vi "Write outgoing label data.vi"(4 "ScheduledSDI":bool, 6 "Iteration":i32, 8 "error in (no error)":errorcluster, 9 "Last iteration values":dbl[](array[numeric]), 10 "This iteration values":dbl[](array[numeric]), 11 "Label Settings":T1 {"Words"."Param Setting"."Num Bits" min=1 max=32; "Words"."Param Setting"."Start Bit" min=8 max=31; "Words"."Block Data Refs"."Data Reference" format="%.0x"; "Label" format="%.0o"}) -> (0 "error out":errorcluster, 1 "Last iteration values Out":dbl[](array[numeric]), 3 "Label Settings":T1 {"Words"."Param Setting"."Num Bits" min=1 max=32; "Words"."Param Setting"."Start Bit" min=8 max=31; "Words"."Block Data Refs"."Data Reference" format="%.0x"; "Label" format="%.0o"})   [LabVIEW 2012, in "AIT 429 Engine.lvlib"]
uses:
  AIT 429 Engine.lvlib
  RT Controls/RT Label Settings.ctl
  Shared/Controls and Global/Label.ctl
  Shared/Controls and Global/transferPeriod.ctl
  RT Controls/Driver Data.ctl
  RT Controls/RT Word Settings.ctl
  <vilib>/NI Veristand/Custom Device API/Block Data Reference.ctl
  <vilib>/NI Veristand/Custom Device API/Data Reference.ctl
  RT Controls/RT Param Setting.ctl
  Shared/Controls and Global/Start Bit.ctl
  Shared/Controls and Global/Number of Bits.ctl
  Shared/Controls and Global/TransferType.ctl
  <instrlib>/AIT 429/AIT 429.lvlib
  ARINC 429 Shared.lvlib
  <vilib>/NI Veristand/Custom Device API/Custom Device API.lvlib
panel:
  in  "Array length":i32
  in  "Array index":i32
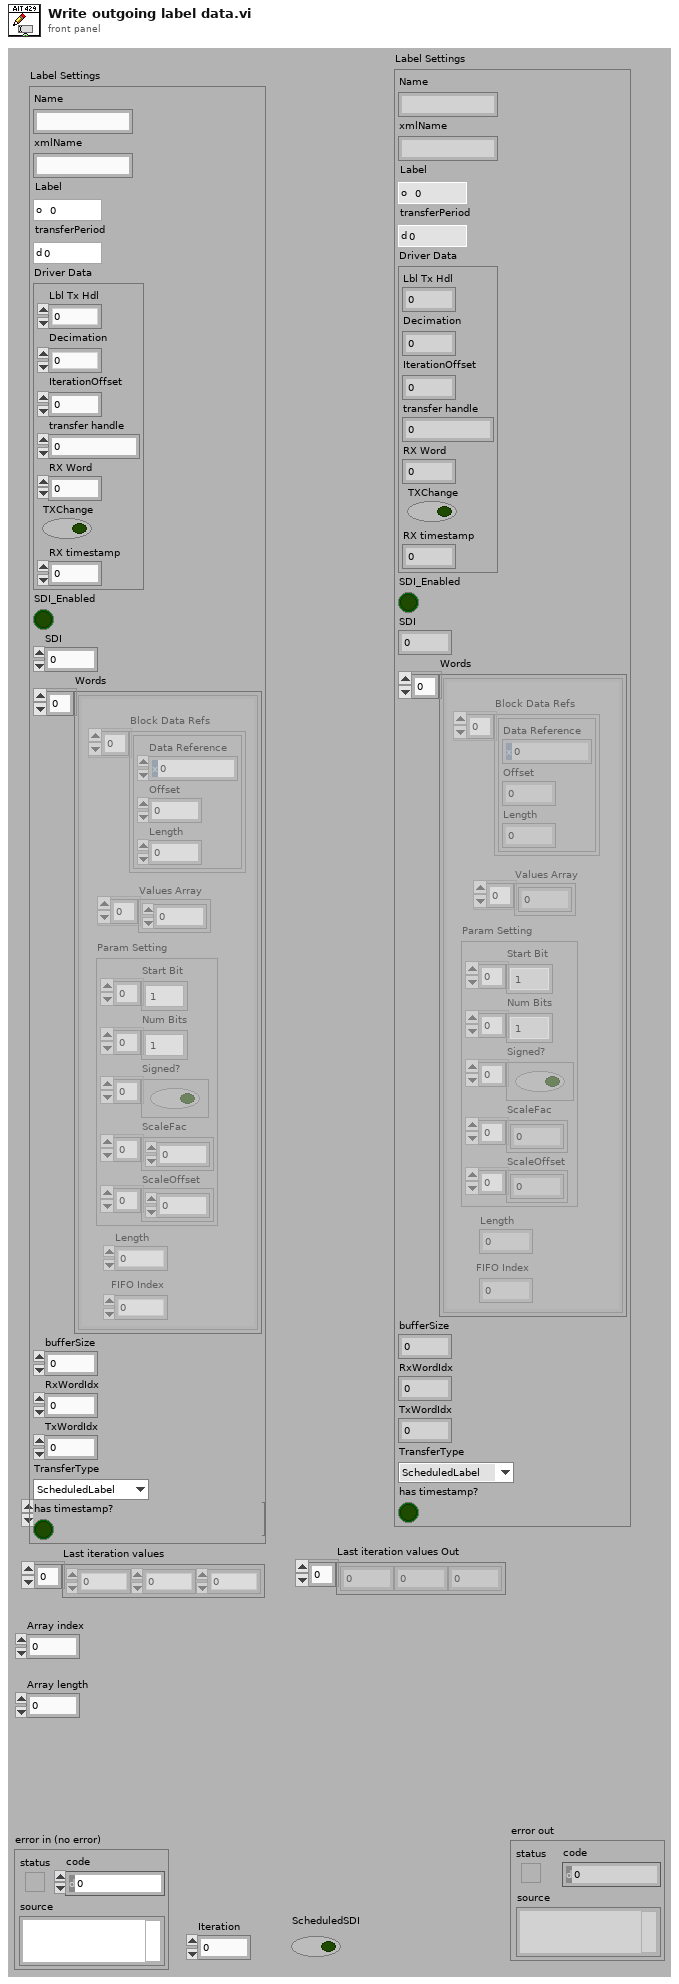
[diagram p1: front panel]
types:
  T1 = typedef "AIT 429 Engine.lvlib/RT Label Settings.ctl" = cluster{"Name":string, "xmlName":string, "Label":T2, "transferPeriod":T3, "Driver Data":T4, "SDI_Enabled":bool, "SDI":u8, "Words":T5[], "bufferSize":u32, "RxWordIdx":i32, "TxWordIdx":i32, "TransferType":T11, "has timestamp?":bool}
  T2 = typedef "ARINC 429 Shared.lvlib/Label.ctl" = u8
  T3 = typedef "ARINC 429 Shared.lvlib/transferPeriod.ctl" = u32
  T4 = typedef "AIT 429 Engine.lvlib/Driver Data.ctl" = cluster{"Lbl Tx Hdl":u32, "Decimation":i32, "IterationOffset":i32, "transfer handle":u32, "RX Word":u32, "TXChange":bool, "RX timestamp":dbl}
  T5 = typedef "AIT 429 Engine.lvlib/RT Word Settings.ctl" = cluster{"Block Data Refs":T6[], "Values Array":dbl[], "Length":i32, "FIFO Index":i32, "Param Setting":T8}
  T6 = typedef "Custom Device API.lvlib/Block Data Reference.ctl" = cluster{"Data Reference":T7, "Offset":i32, "Length":i32}
  T7 = typedef "Custom Device API.lvlib/Data Reference.ctl" = i32
  T8 = typedef "AIT 429 Engine.lvlib/RT Param Setting.ctl" = cluster{"Start Bit":T9[], "Num Bits":T10[], "Signed?":bool[], "ScaleFac":dbl[], "ScaleOffset":dbl[]}
  T9 = typedef "ARINC 429 Shared.lvlib/Start Bit.ctl" = i32
  T10 = typedef "ARINC 429 Shared.lvlib/Number of Bits.ctl" = i32
  T11 = typedef "ARINC 429 Shared.lvlib/TransferType.ctl" = enum16{"ScheduledLabel", "Acyclic", "Block", "Strobe"}
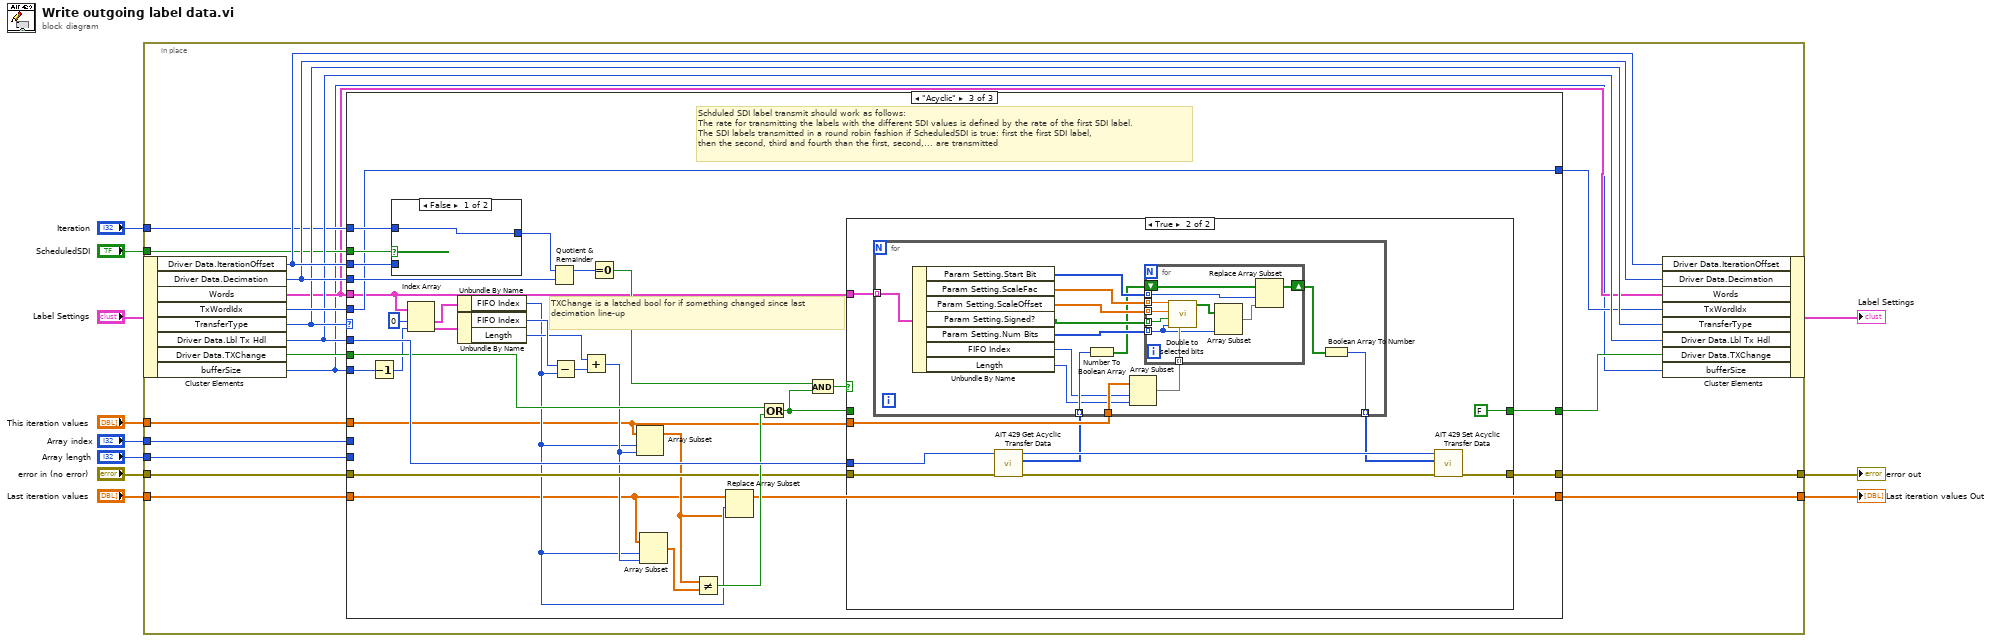
[diagram p0: block diagram]
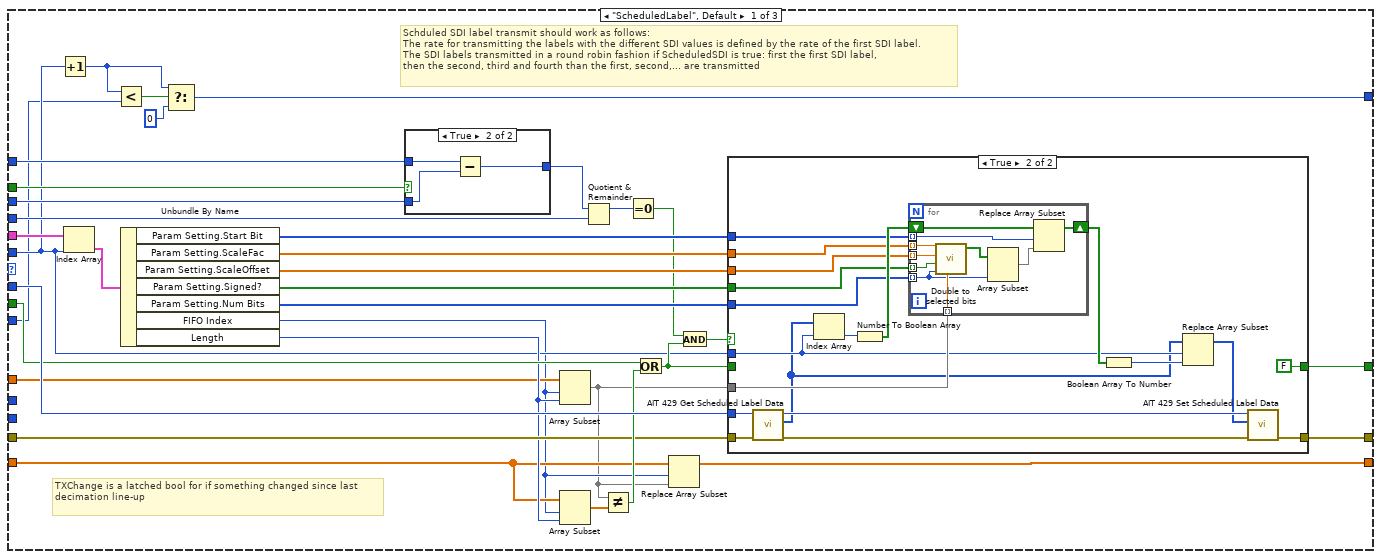
[diagram p2: hidden frame]
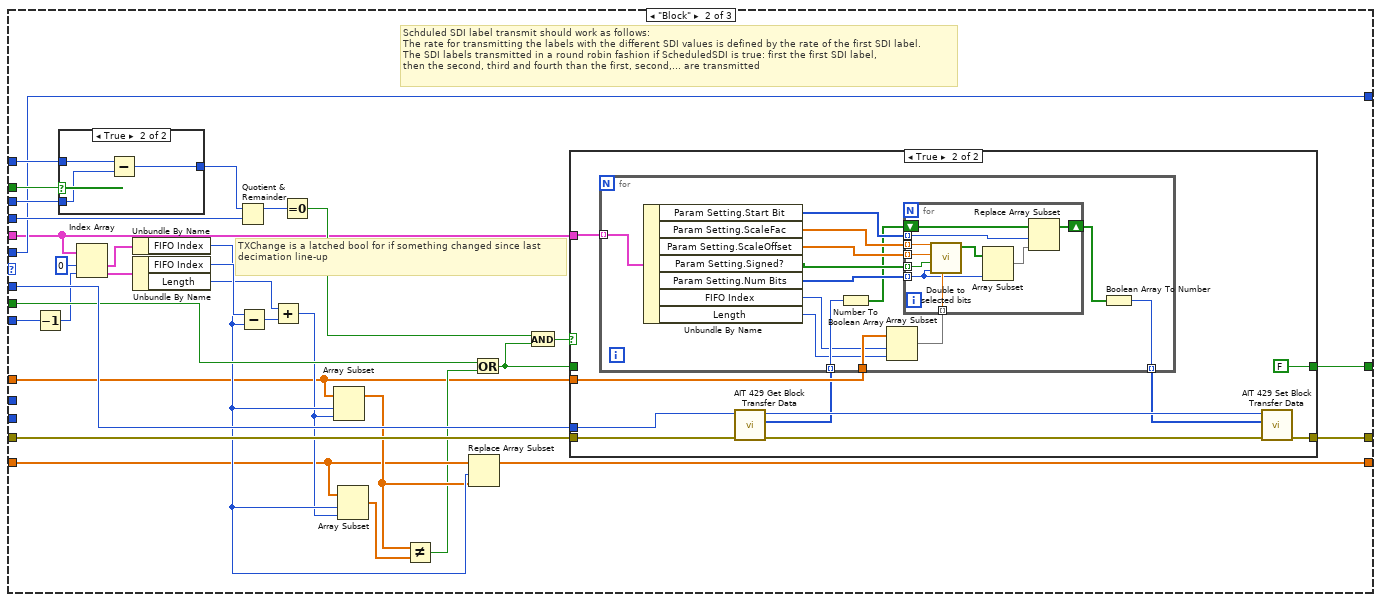
[diagram p5: hidden frame]
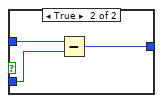
[diagram p9: hidden frame]
diagram:
  n1 = in-place {
    in-place-border: "This iteration values" -> [w27]
    in-place-border: "Array index" -> [w26]
    in-place-border: "Array length" -> [w25]
    in-place-border: "error in (no error)" -> [w24]
    in-place-border: "Last iteration values" -> [w23]
    in-place-border: [w22] -> w5
    in-place-border: "Iteration" -> [w17]
    in-place-border: "ScheduledSDI" -> [w16]
    in-place-border: [w13] -> w1
    n2 = in-place-cluster #1("Label Settings") -> ("Driver Data.IterationOffset"=w21:i32, "Driver Data.Decimation"=w20:i32, "Words"=w14:T5[], "TxWordIdx"=w30:i32, "TransferType"=w19:T11, "Driver Data.Lbl Tx Hdl"=w18:u32, "Driver Data.TXChange"=w29:bool, "bufferSize"=w12:u32)
    n3 = case shown="\"Acyclic\"" w19 {
      tunnel: w30 -> [w36 w118 w189]
      tunnel: w14 -> [w65 w117 w188]
      tunnel: w21 -> [w64 w132 w204]
      tunnel: w20 -> [w63 w131 w203]
      tunnel: w18 -> [w62 w130 w202]
      tunnel: w29 -> [w61 w129 w201]
      tunnel: [w60 w128 w200] -> w28
      tunnel: w27 -> [w38 w101 w173]
      tunnel: w26 -> [_ _ _]
      tunnel: w25 -> [_ _ _]
      tunnel: w24 -> [w47 w122 w193]
      tunnel: w23 -> [w34 w104 w174]
      tunnel: [w46 w121 w192] -> w22
      tunnel: w17 -> [w45 w120 w191]
      tunnel: w16 -> [w44 w119 w190]
      tunnel: [w41 w118 w189] -> w15
      tunnel: [w35 w108 w178] -> w13
      tunnel: w12 -> [w31 w115 w186]
      frame "ScheduledLabel", Default {
        # "TXChange is a latched bool for if something changed since last decimation line-up"
        # "Schduled SDI label transmit should work as follows:\nThe rate for transmitting the labels with the different SDI values is defined by the rate of the first SDI label.\nThe SDI labels transmitted in a round robin fashion if ScheduledSDI is true: first the first SDI label, \nthen the second, third and fourth than the first, second,... are transmitted"
        n4 = Increment(x=w36) -> (x+1=w39:i32)
        n5 = Index Array(array=w65, index=w36) -> (element=w59:T5)
        n6 = Less?(x=w39, y=w31) -> (x < y?=w43:bool)
        n7 = Unbundle By Name(w59) -> ("Param Setting.Start Bit"=w58:T9[], "Param Setting.ScaleFac"=w57:dbl[], "Param Setting.ScaleOffset"=w56:dbl[], "Param Setting.Signed?"=w55:bool[], "Param Setting.Num Bits"=w54:T10[], "FIFO Index"=w33:i32, "Length"=w40:i32)
        n8 = Select(t=w39, s=w43, f=0 ("TxWordIdx")) -> (s? t:f=w41:i32)
        n9 = case shown="True" w44 {
          tunnel: w45 -> [w97 w98]
          tunnel: [w97 w100] -> w52
          tunnel: w64 -> [_ w99]
          frame False {
          }
          frame True {
            n10 = Subtract(x=w98, y=w99) -> (x-y=w100:i32)
          }
        }
        n11 = Array Subset(array=w38, index=w33, length=w40) -> (w32:dbl[])
        n12 = Array Subset(array=w34, index=w33, length=w40) -> (w37:dbl[])
        n13 = Quotient & Remainder(x=w52, y=w63) -> (x-y*floor(x/y)=w53:i32)  [unwired: 1 out]
        n14 = Not Equal?(x=w32, y=w37) -> (x != y?=w51:bool)
        n15 = Equal To 0?(x=w53) -> (x = 0?=w50:bool)
        n16 = Or(x=w61, y=w51) -> (x .or. y?=w48:bool)
        n17 = Replace Array Subset(array=w34, new element=w32, index=w33) -> (w35:dbl[])
        n18 = And(x=w50, y=w48) -> (x .and. y?=w49:bool)
        n19 = case shown="True" w49 {
          tunnel: w58 -> [_ w83]
          tunnel: w54 -> [_ w84]
          tunnel: [w67 w74] -> w46
          tunnel: w47 -> [w67 w78]
          tunnel: w62 -> [_ w77]
          tunnel: w57 -> [_ w82]
          tunnel: w56 -> [_ w81]
          tunnel: w55 -> [_ w80]
          tunnel: w32 -> [_ w79]
          tunnel: w48 -> [w66 _]
          tunnel: [w66 FALSE] -> w60
          tunnel: w36 -> [_ w71]
          frame False {
          }
          frame True {
            (unwired) FALSE
            n20 = call <instrlib>:"AIT 429 Get Scheduled Label Data.vi"("error in (no error)"=w78, "scheduled label handle"=w77) -> ("error out"=w75:errorcluster, "word array"=w70:u32[], "scheduled label handle"=w73:u32)  [unwired: 7 in]
            n21 = Index Array(array=w70, index=w71) -> (element=w76:u32)
            n22 = Number To Boolean Array(number=w76) -> (Boolean array=w86:bool[])
            n23 = for {
              tunnel: w83 -> [w95] mode=indexing
              tunnel: w84 -> [w90] mode=indexing
              tunnel: w79 -> [w91] mode=indexing
              shift-right: [w93] -> w85
              shift-left: w86 -> [w96]
              tunnel: w82 -> [w89] mode=indexing
              tunnel: w81 -> [w88] mode=indexing
              tunnel: w80 -> [w87] mode=indexing
              n24 = call "Double to selected bits.vi"("Double"=w91, "Number of Bits"=w90, "Signed?"=w87, "ScaleOffset"=w88, "ScaleFac"=w89) -> ("Bits"=w92:bool[])  [unwired: 6 in]
              n25 = Array Subset(array=w92, length=w90) -> (w94:bool[])  [unwired: 1 in]
              n26 = Replace Array Subset(array=w96, new element=w94, index=w95) -> (w93:bool[])
            }
            n27 = Boolean Array To Number(Boolean array=w85) -> (number=w72:u32)
            n28 = Replace Array Subset(array=w70, new element=w72, index=w71) -> (w69:u32[])
            n29 = call <instrlib>:"AIT 429 Set Scheduled Label Data.vi"("error in (no error)"=w75, "word array"=w69, "scheduled label handle"=w73) -> ("error out"=w74:errorcluster)  [unwired: 6 in, 2 out]
          }
        }
      }
      frame "Block" {
        # "TXChange is a latched bool for if something changed since last decimation line-up"
        # "Schduled SDI label transmit should work as follows:\nThe rate for transmitting the labels with the different SDI values is defined by the rate of the first SDI label.\nThe SDI labels transmitted in a round robin fashion if ScheduledSDI is true: first the first SDI label, \nthen the second, third and fourth than the first, second,... are transmitted"
        n30 = Decrement(x=w115) -> (x-1=w114:u32)
        n31 = case shown="True" w119 {
          tunnel: w120 -> [w169 w170]
          tunnel: [w169 w172] -> w126
          tunnel: w132 -> [_ w171]
          frame False {
          }
          frame True {
            n32 = Subtract(x=w170, y=w171) -> (x-y=w172:i32)
          }
        }
        n33 = Index Array(array=w117, index #1=0 ("index"), index #2=w114) -> (element #1=w113:T5, element #2=w112:T5)
        n34 = Unbundle By Name(w113) -> ("FIFO Index"=w107:i32)
        n35 = Unbundle By Name(w112) -> ("FIFO Index"=w111:i32, "Length"=w109:i32)
        n36 = Quotient & Remainder(x=w126, y=w131) -> (x-y*floor(x/y)=w127:i32)  [unwired: 1 out]
        n37 = Subtract(x=w111, y=w107) -> (x-y=w110:i32)
        n38 = Add(x=w109, y=w110) -> (x+y=w106:i32)
        n39 = Equal To 0?(x=w127) -> (x = 0?=w125:bool)
        n40 = Array Subset(array=w101, index=w107, length=w106) -> (w105:dbl[])
        n41 = Array Subset(array=w104, index=w107, length=w106) -> (w103:dbl[])
        n42 = Not Equal?(x=w105, y=w103) -> (x != y?=w102:bool)
        n43 = Replace Array Subset(array=w104, new element=w105, index=w107) -> (w108:dbl[])
        n44 = Or(x=w129, y=w102) -> (x .or. y?=w123:bool)
        n45 = And(x=w125, y=w123) -> (x .and. y?=w124:bool)
        n46 = case shown="True" w124 {
          tunnel: [w134 w139] -> w121
          tunnel: w122 -> [w134 w141]
          tunnel: w130 -> [_ w138]
          tunnel: w101 -> [_ w142]
          tunnel: w123 -> [w133 _]
          tunnel: [w133 FALSE] -> w128
          tunnel: w117 -> [_ w143]
          frame False {
          }
          frame True {
            n47 = call <instrlib>:"AIT 429 Get Block Transfer Data.vi"("error in"=w141, "block transfer handle in"=w138) -> ("error out"=w140:errorcluster, "word array out"=w136:u32[], "block transfer handle out"=w137:u32)  [unwired: 7 in]
            n48 = for {
              tunnel: w142 -> [w148]
              tunnel: [w157] -> w135 mode=indexing
              tunnel: w143 -> [w151] mode=indexing
              tunnel: w136 -> [w149] mode=indexing
              n49 = Unbundle By Name(w151) -> ("Param Setting.Start Bit"=w156:T9[], "Param Setting.ScaleFac"=w155:dbl[], "Param Setting.ScaleOffset"=w154:dbl[], "Param Setting.Signed?"=w153:bool[], "Param Setting.Num Bits"=w152:T10[], "FIFO Index"=w147:i32, "Length"=w146:i32)
              n50 = Number To Boolean Array(number=w149) -> (Boolean array=w150:bool[])
              n51 = Array Subset(array=w148, index=w147, length=w146) -> (w145:dbl[])
              n52 = for {
                tunnel: w156 -> [w167] mode=indexing
                tunnel: w152 -> [w162] mode=indexing
                tunnel: w145 -> [w163] mode=indexing
                shift-right: [w165] -> w158
                shift-left: w150 -> [w168]
                tunnel: w155 -> [w161] mode=indexing
                tunnel: w154 -> [w160] mode=indexing
                tunnel: w153 -> [w159] mode=indexing
                n53 = call "Double to selected bits.vi"("Double"=w163, "Number of Bits"=w162, "Signed?"=w159, "ScaleOffset"=w160, "ScaleFac"=w161) -> ("Bits"=w164:bool[])  [unwired: 6 in]
                n54 = Array Subset(array=w164, length=w162) -> (w166:bool[])  [unwired: 1 in]
                n55 = Replace Array Subset(array=w168, new element=w166, index=w167) -> (w165:bool[])
              }
              n56 = Boolean Array To Number(Boolean array=w158) -> (number=w157:u32)
            }
            n57 = call <instrlib>:"AIT 429 Set Block Transfer Data.vi"("error in (no error)"=w140, "word array"=w135, "block transfer handle in"=w137) -> ("error out"=w139:errorcluster)  [unwired: 6 in, 2 out]
          }
        }
      }
      frame "Acyclic" {
        # "TXChange is a latched bool for if something changed since last decimation line-up"
        # "Schduled SDI label transmit should work as follows:\nThe rate for transmitting the labels with the different SDI values is defined by the rate of the first SDI label.\nThe SDI labels transmitted in a round robin fashion if ScheduledSDI is true: first the first SDI label, \nthen the second, third and fourth than the first, second,... are transmitted"
        n58 = Decrement(x=w186) -> (x-1=w185:u32)
        n59 = case shown="False" w190 {
          tunnel: w191 -> [w241 w242]
          tunnel: [w241 w244] -> w198
          tunnel: w204 -> [_ w243]
          frame False {
          }
          frame True {
            n60 = Subtract(x=w242, y=w243) -> (x-y=w244:i32)
          }
        }
        n61 = Index Array(array=w188, index #1=0 ("index"), index #2=w185) -> (element #1=w184:T5, element #2=w183:T5)
        n62 = Unbundle By Name(w184) -> ("FIFO Index"=w177:i32)
        n63 = Unbundle By Name(w183) -> ("FIFO Index"=w182:i32, "Length"=w180:i32)
        n64 = Quotient & Remainder(x=w198, y=w203) -> (x-y*floor(x/y)=w199:i32)  [unwired: 1 out]
        n65 = Subtract(x=w182, y=w177) -> (x-y=w181:i32)
        n66 = Add(x=w180, y=w181) -> (x+y=w179:i32)
        n67 = Equal To 0?(x=w199) -> (x = 0?=w196:bool)
        n68 = Array Subset(array=w173, index=w177, length=w179) -> (w176:dbl[])
        n69 = Array Subset(array=w174, index=w177, length=w179) -> (w175:dbl[])
        n70 = Not Equal?(x=w176, y=w175) -> (x != y?=w197:bool)
        n71 = Replace Array Subset(array=w174, new element=w176, index=w177) -> (w178:dbl[])
        n72 = Or(x=w201, y=w197) -> (x .or. y?=w194:bool)
        n73 = And(x=w196, y=w194) -> (x .and. y?=w195:bool)
        n74 = case shown="True" w195 {
          tunnel: [w206 w208] -> w192
          tunnel: w193 -> [w206 w210]
          tunnel: w202 -> [_ w213]
          tunnel: w173 -> [_ w214]
          tunnel: w194 -> [w205 _]
          tunnel: [w205 FALSE] -> w200
          tunnel: w188 -> [_ w215]
          frame False {
          }
          frame True {
            n75 = call <instrlib>:"AIT 429 Get Acyclic Transfer Data.vi"("error in (no error)"=w210, "transfer handle"=w213) -> ("error out"=w209:errorcluster, "word array"=w211:u32[], "transfer handle"=w212:u32)  [unwired: 7 in]
            n76 = for {
              tunnel: w214 -> [w220]
              tunnel: [w229] -> w207 mode=indexing
              tunnel: w215 -> [w223] mode=indexing
              tunnel: w211 -> [w221] mode=indexing
              n77 = Unbundle By Name(w223) -> ("Param Setting.Start Bit"=w228:T9[], "Param Setting.ScaleFac"=w227:dbl[], "Param Setting.ScaleOffset"=w226:dbl[], "Param Setting.Signed?"=w225:bool[], "Param Setting.Num Bits"=w224:T10[], "FIFO Index"=w219:i32, "Length"=w218:i32)
              n78 = Number To Boolean Array(number=w221) -> (Boolean array=w222:bool[])
              n79 = Array Subset(array=w220, index=w219, length=w218) -> (w217:dbl[])
              n80 = for {
                tunnel: w228 -> [w239] mode=indexing
                tunnel: w224 -> [w234] mode=indexing
                tunnel: w217 -> [w235] mode=indexing
                shift-right: [w237] -> w230
                shift-left: w222 -> [w240]
                tunnel: w227 -> [w233] mode=indexing
                tunnel: w226 -> [w232] mode=indexing
                tunnel: w225 -> [w231] mode=indexing
                n81 = call "Double to selected bits.vi"("Double"=w235, "Number of Bits"=w234, "Signed?"=w231, "ScaleOffset"=w232, "ScaleFac"=w233) -> ("Bits"=w236:bool[])  [unwired: 6 in]
                n82 = Array Subset(array=w236, length=w234) -> (w238:bool[])  [unwired: 1 in]
                n83 = Replace Array Subset(array=w240, new element=w238, index=w239) -> (w237:bool[])
              }
              n84 = Boolean Array To Number(Boolean array=w230) -> (number=w229:u32)
            }
            n85 = call <instrlib>:"AIT 429 Set Acyclic Transfer Data.vi"("error in (no error)"=w209, "word array"=w207, "transfer handle"=w212) -> ("error out"=w208:errorcluster)  [unwired: 7 in, 1 out]
          }
        }
      }
    }
    n86 = in-place-cluster #1("Driver Data.IterationOffset"=w21, "Driver Data.Decimation"=w20, "Words"=w14, "TxWordIdx"=w15, "TransferType"=w19, "Driver Data.Lbl Tx Hdl"=w18, "Driver Data.TXChange"=w28, "bufferSize"=w12) -> (→"Label Settings":T1)
  }
  "error out" <- w5
  "Last iteration values Out" <- w1
